vi "HeaderFileCheck.vi"(11 "result string in":string) -> (2 "Integration time":dbl, 3 "result string out":string)   [LabVIEW 2020]
uses:
  <vilib>/regexp/Match Regular Expression.xnode
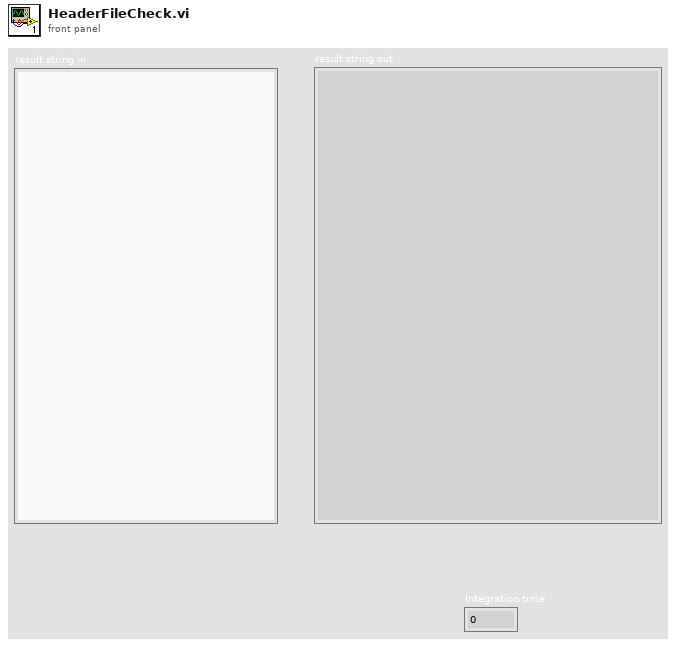
[diagram p1: front panel]
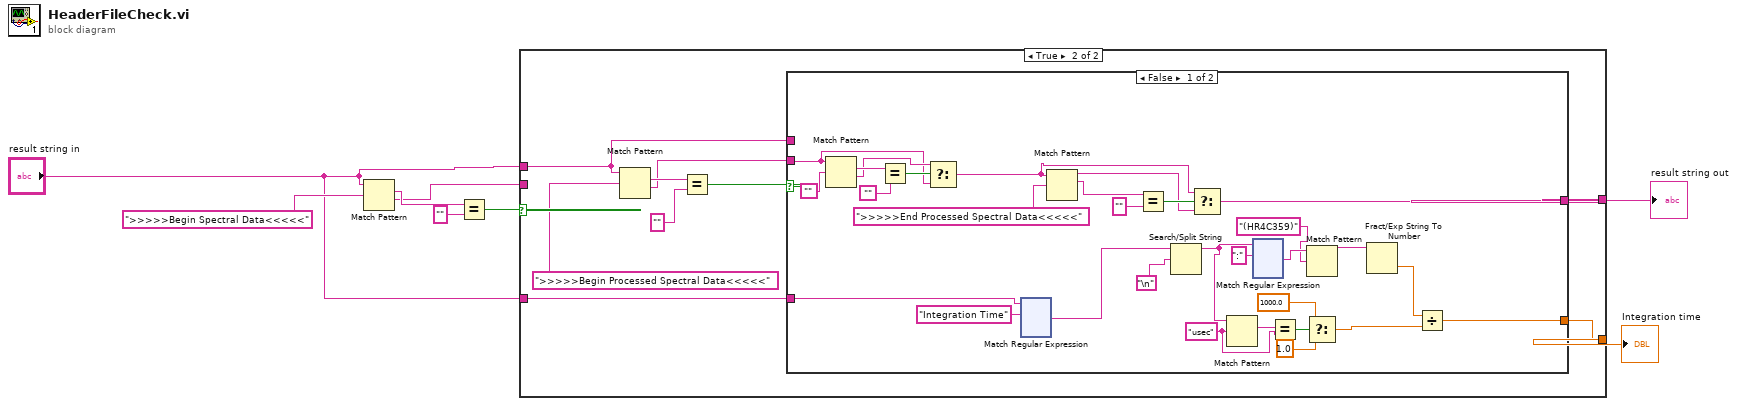
[diagram p0: block diagram]
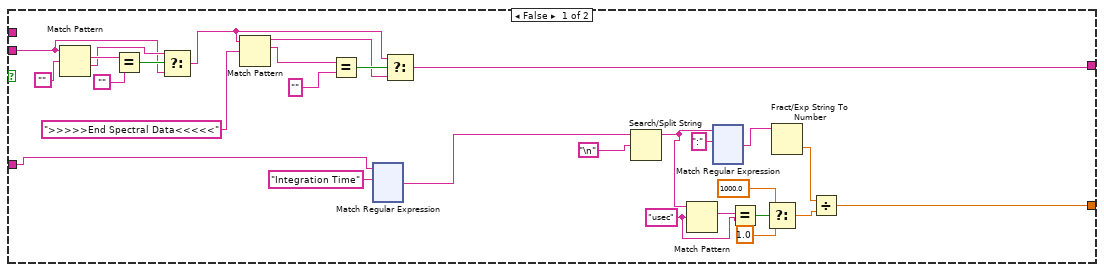
[diagram p2: hidden frame]
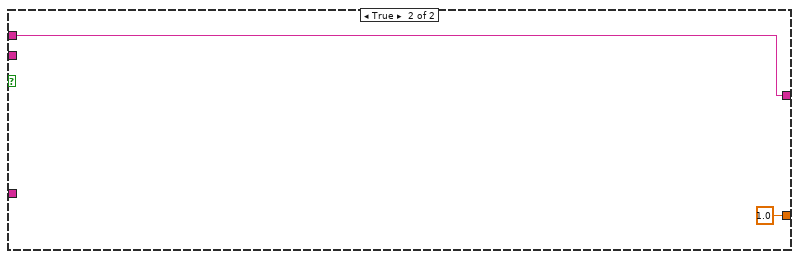
[diagram p3: hidden frame]
diagram:
  n1 = Match Pattern(string="result string in", regular expression=">>>>>Begin Spectral Data<<<<<") -> (match substring=w7:string, after substring=w2:string)  [unwired: 1 in, 2 out]
  n2 = Equal?(x=w7, y="") -> (x = y?=w5:bool)
  n3 = case shown="True" w5 {
    tunnel: "result string in" -> [_ w267]
    tunnel: [w19 w268] -> w4
    tunnel: [w18 w269] -> w3
    tunnel: w2 -> [w10 _]
    tunnel: "result string in" -> [w16 w265]
    frame False {
      w27 = "usec" ("regular expression")
      n4 = Match Pattern(string=w10, regular expression="") -> (match substring=w14:string, after substring=w11:string)  [unwired: 1 in, 2 out]
      n5 = Equal?(x=w14, y="") -> (x = y?=w12:bool)
      n6 = Select(t=w11, s=w12, f=w10) -> (s? t:f=w9:string)
      n7 = Match Pattern(string=w9, regular expression=">>>>>End Spectral Data<<<<<") -> (before substring=w17:string, match substring=w34:string)  [unwired: 1 in, 2 out]
      n8 = Equal?(x=w34, y="") -> (x = y?=w35:bool)
      n9 = xnode "Match Regular Expression"("input string"=w16, "regular expression"="Integration Time") -> ("after match"=w21:string)  [unwired: 4 in, 4 out]
      n10 = Select(t=w9, s=w35, f=w17) -> (s? t:f=w18:string)
      n11 = Search/Split String(string=w21, search string/char (-)="\n") -> (substring before match=w22:string)  [unwired: 1 in, 2 out]
      n12 = Match Pattern(string=w22, regular expression=w27) -> (match substring=w26:string)  [unwired: 1 in, 3 out]
      n13 = xnode "Match Regular Expression"("input string"=w22, "regular expression"=":") -> ("after match"=w20:string)  [unwired: 4 in, 4 out]
      n14 = Equal?(x=w26, y=w27) -> (x = y?=w28:bool)
      n15 = Select(t=1000.0, s=w28, f=1.0) -> (s? t:f=w32:dbl)
      n16 = Fract/Exp String To Number(string=w20) -> (number=w31:dbl)  [unwired: 3 in, 1 out]
      n17 = Divide(x=w31, y=w32) -> (x/y=w19:dbl)
    }
    frame True {
      n18 = Match Pattern(string=w267, regular expression=">>>>>Begin Processed Spectral Data<<<<<") -> (match substring=w270:string, after substring=w266:string)  [unwired: 1 in, 2 out]
      n19 = Equal?(x=w270, y="") -> (x = y?=w271:bool)
      n20 = case shown="False" w271 {
        tunnel: [w299 w533] -> w269
        tunnel: [w283 1.0] -> w268
        tunnel: w267 -> [_ w533]
        tunnel: w266 -> [w275 _]
        tunnel: w265 -> [w281 _]
        frame False {
          w293 = "usec" ("regular expression")
          n21 = Match Pattern(string=w275, regular expression="") -> (match substring=w279:string, after substring=w276:string)  [unwired: 1 in, 2 out]
          n22 = Equal?(x=w279, y="") -> (x = y?=w277:bool)
          n23 = Select(t=w276, s=w277, f=w275) -> (s? t:f=w274:string)
          n24 = xnode "Match Regular Expression"("input string"=w281, "regular expression"="Integration Time") -> ("after match"=w287:string)  [unwired: 4 in, 4 out]
          n25 = Match Pattern(string=w274, regular expression=">>>>>End Processed Spectral Data<<<<<") -> (before substring=w282:string, match substring=w301:string)  [unwired: 1 in, 2 out]
          n26 = Equal?(x=w301, y="") -> (x = y?=w302:bool)
          n27 = Search/Split String(string=w287, search string/char (-)="\n") -> (substring before match=w288:string)  [unwired: 1 in, 2 out]
          n28 = Select(t=w274, s=w302, f=w282) -> (s? t:f=w299:string)
          n29 = Match Pattern(string=w288, regular expression=w293) -> (match substring=w292:string)  [unwired: 1 in, 3 out]
          n30 = xnode "Match Regular Expression"("input string"=w288, "regular expression"=":") -> ("after match"=w286:string)  [unwired: 4 in, 4 out]
          n31 = Equal?(x=w292, y=w293) -> (x = y?=w294:bool)
          n32 = Match Pattern(string=w286, regular expression="(HR4C359)" ("string")) -> (before substring=w284:string)  [unwired: 1 in, 3 out]
          n33 = Select(t=1000.0, s=w294, f=1.0) -> (s? t:f=w298:dbl)
          n34 = Fract/Exp String To Number(string=w284) -> (number=w297:dbl)  [unwired: 3 in, 1 out]
          n35 = Divide(x=w297, y=w298) -> (x/y=w283:dbl)
        }
        frame True {
        }
      }
    }
  }
  "result string out" <- w3
  "Integration time" <- w4
